vi "AlazarDSPGetInfo.vi"(0 "DSP Handle":u64, 11 "error in (no error)":errorcluster) -> (1 "Module ID":u32, 2 "Version Major":u16, 3 "Version Minor":u16, 4 "DSP Handle":u64, 6 "Max Length":u32, 10 "Return Code":u32, 13 "Reserved 1":u32, 14 "Reserved 0":u32, 15 "error out":errorcluster)   [LabVIEW 2018]
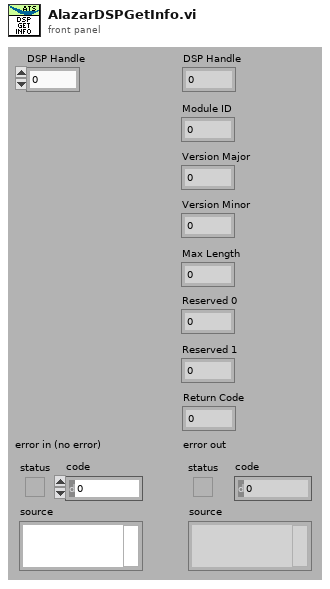
[diagram p1: front panel]
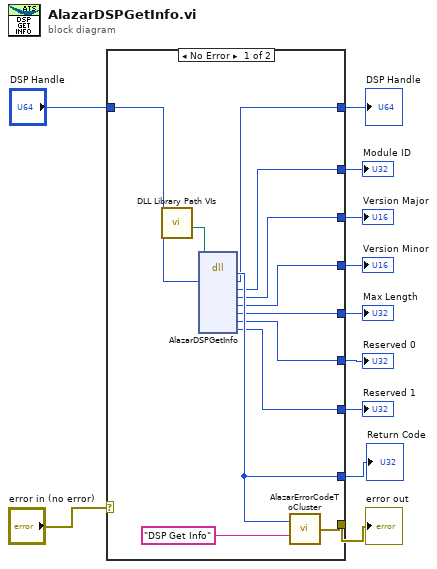
[diagram p0: block diagram]
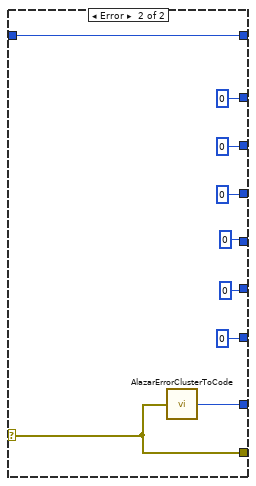
[diagram p2: hidden frame]
diagram:
  n1 = case shown="No Error" "error in (no error)" {
    selector: "error in (no error)" -> [_ w32]
    tunnel: [w20 w32] -> w10
    tunnel: [w22 w31] -> w9
    tunnel: "DSP Handle" -> [w23 w30]
    tunnel: [w19 w30] -> w7
    tunnel: [w18 0] -> w6
    tunnel: [w17 0] -> w5
    tunnel: [w16 0] -> w4
    tunnel: [w15 0] -> w3
    tunnel: [w14 0] -> w2
    tunnel: [w13 0] -> w1
    frame No Error {
      n2 = call "DLL Library Path VIs.vi"() -> ("Alazar"=w12:path)  [unwired: 9 in, 2 out]
      n3 = dll-call lib="C:/Project/SerialSectOCT - FFT GPU/SerialSectOCT/Labview Software/DLL/ATSApi.dll" fn="AlazarDSPGetInfo"(path in=w12, "handle"=w23) -> ("return type"=w22:u32, "handle"=w19:u64, "moduleId"=w18:u32, "versionMajor"=w17:u16, "versionMinor"=w16:u16, "maxLength"=w15:u32, "Reserved 0"=w14:u32, "Reserved 1"=w13:u32)  [unwired: 8 in, 2 out]
      n4 = call "AlazarErrorCodeToCluster.vi"("Message"="DSP Get Info", "Error Code"=w22) -> ("error out"=w20:errorcluster)
    }
    frame Error {
      n5 = call "AlazarErrorClusterToCode.vi"("error in (no error)"=w32) -> ("Error Code"=w31:u32)
    }
  }
  "DSP Handle" <- w7
  "error out" <- w10
  "Return Code" <- w9
  "Module ID" <- w6
  "Version Major" <- w5
  "Version Minor" <- w4
  "Max Length" <- w3
  "Reserved 0" <- w2
  "Reserved 1" <- w1
